vi "Initialise.vi"(8 "error in (no error)":errorcluster, 10 "Message in":refnum<class "InitialiseMessage.lvclass">, 11 "AOTF in":refnum<class "AOTF.lvclass">) -> (0 "error out":errorcluster, 3 "AOTF out":refnum<class "AOTF.lvclass">)   [LabVIEW 2012, in "AOTF.lvclass"]
doc: "This method is called when an initialise message is received. It mainly initialises the RabbitMQ connectivity. \n\nOverride this method when your component needs special initialisation (e.g. of software or hardware resources). In that case, don't forget to call the parent for proper implementation. If your component owns subcomponents, they count as resources, so you have to initialise them by calling their own initialise functions"
uses:
  AOTF.lvclass
  <vilib>/Distrio/Murmex/InitialiseMessage/InitialiseMessage.lvclass
  <vilib>/Distrio/Murmex/Murmex/Murmex.lvclass
  AOTF.lvclass/AOTF.ctl
  <vilib>/DAQmx/create/channels.llb/DAQmx Create Channel (DO-Digital Output).vi
  <vilib>/DAQmx/create/channels.llb/DAQmx Create Channel (AO-Voltage-Basic).vi
panel:
  # "This method is called when the INTIALISE\ntrigger is sent. \n\nOverride this method when your component needs to\nrespond to this trigger. \n\nCall parent for proper implementation"
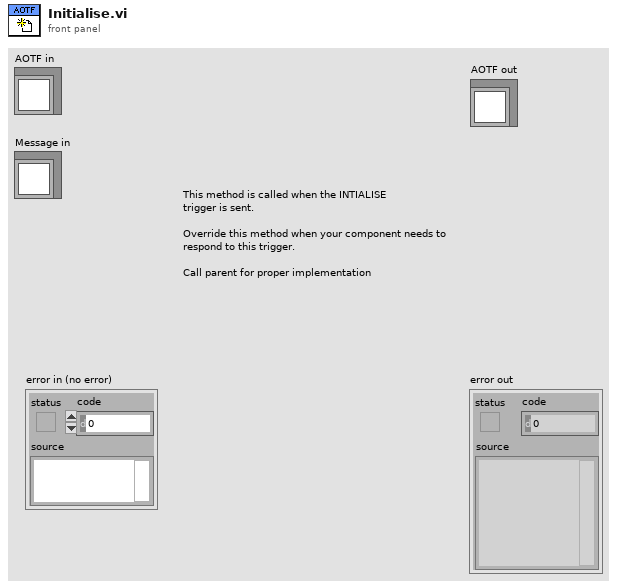
[diagram p1: front panel]
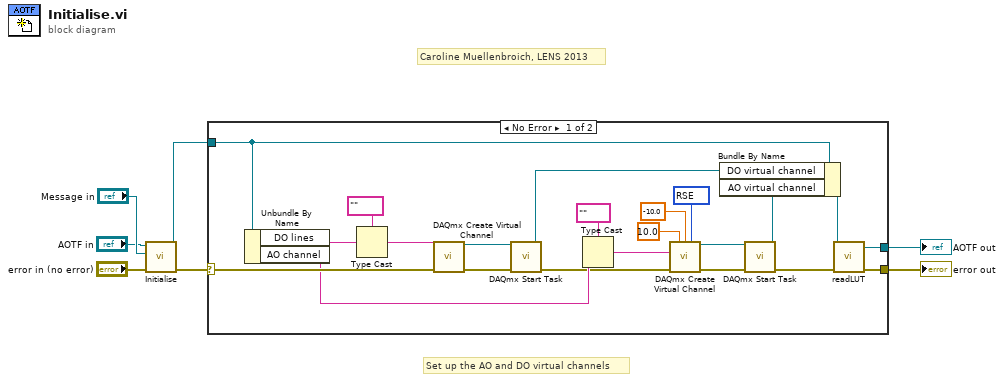
[diagram p0: block diagram]
diagram:
  # "Set up the AO and DO virtual channels"
  # "Caroline Muellenbroich, LENS 2013"
  n1 = call-parent "Initialise.vi"("error in (no error)"="error in (no error)", "Message in"="Message in", "Murmex in"="AOTF in") -> ("error out"=w4:errorcluster, "Murmex out"=w3:refnum<class "AOTF.lvclass">)  [unwired: 7 in]
  n2 = case shown="No Error" w4 {
    selector: w4 -> [w25 w31]
    tunnel: w3 -> [w26 w30]
    tunnel: [w29 w31] -> w2
    tunnel: [w27 w30] -> w1
    frame No Error {
      w24 = 10083 items=["Default"=-1, "RSE"=10083, "Differential"=10106, "Pseudodifferential"=12529] ("output terminal configuration")
      n3 = Unbundle By Name(w26) -> ("DO lines"=w17:string, "AO channel"=w12:string)
      n4 = Type Cast(type=tag "" ("lines"), x=w17) -> (*(type *) &x=w15:tag)
      n5 = call-poly <vilib>:"DAQmx Create Virtual Channel.vi"("lines"=w15, "error in"=w25) -> ("task out"=w20:refnum<k21>, "error out"=w21:errorcluster)  [unwired: 12 in]
      n6 = call <vilib>:"DAQmx Start Task.vi"("task/channels in"=w20, "error in"=w21) -> ("task out"=w10:refnum<k21>, "error out"=w11:errorcluster)  [unwired: 12 in]
      n7 = Type Cast(type=tag "" ("physical channels"), x=w12) -> (*(type *) &x=w13:tag)
      n8 = call-poly <vilib>:"DAQmx Create Virtual Channel.vi"("maximum value"=10.0, "minimum value"=-10.0, "output terminal configuration"=w24, "physical channels"=w13, "error in"=w11) -> ("task out"=w18:refnum<k21>, "error out"=w19:errorcluster)  [unwired: 9 in]
      n9 = call <vilib>:"DAQmx Start Task.vi"("task/channels in"=w18, "error in"=w19) -> ("task out"=w9:refnum<k21>, "error out"=w8:errorcluster)  [unwired: 12 in]
      n10 = Bundle By Name(cluster=w26, "DO virtual channel"=w10, "AO virtual channel"=w9) -> (w28:refnum<class "AOTF.lvclass">)
      n11 = call-dynamic "readLUT.vi"("error in (no error)"=w8, "AOTF in"=w28) -> ("error out"=w29:errorcluster, "AOTF out"=w27:refnum<class "AOTF.lvclass">)  [unwired: 8 in]
    }
    frame Error {
    }
  }
  "error out" <- w2
  "AOTF out" <- w1
